vi "Printer Script Trial 1.vi"() -> ()   [LabVIEW 2013]
uses:
  <instrlib>/ZaberTSeries/Public/Utility/Request.ctl
  <instrlib>/ZaberTSeries/ZaberTSeries.lvlib
  <vilib>/MakerHub/LINX/LMH-LINX.lvlib
panel:
  in  "?":T1={"Device Number"=1, "Command"=21, "Data"=-10000, "Response Count"=1} {"Command" items=["Echo"=55, "Home"=1, "Move Absolute"=20, "Move Relative"=21, "Move at Constant Speed"=22, "Renumber"=2, "Restore Settings"=36, "Stop"=23]}
  in  "?":i32=5
  in  "?":T1={"Device Number"=1, "Command"=21, "Data"=-10000, "Response Count"=1} {"Command" items=["Echo"=55, "Home"=1, "Move Absolute"=20, "Move Relative"=21, "Move at Constant Speed"=22, "Renumber"=2, "Restore Settings"=36, "Stop"=23]}
  in  "?":u16
  in  "Select Stage Serial Port \n(COM 10)":refnum<visa-resource-name>
  in  "Select Arduino Serial Port (COM 9)":refnum<visa-resource-name>
  # "Printing Dialogue #1"
  # "Instructions:\n\n1. Select the correct serial ports for the Zaber stage and the Arduino\n\n2. Press the 'Run' arrow at the left of the menu bar. The stage will move forward to accomodate substrate placement. \n\n3. When the substrate has been placed on the stage, click ok in the pop-up dialogue. The stage will then move into place to begin printing. \n\n4. Click OK the 'Begin Printing' pop-up."
  # "Device 1:"
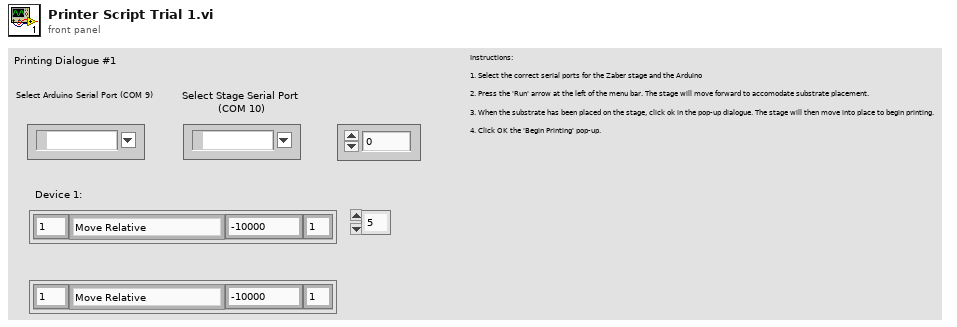
[diagram p1: front panel]
types:
  T1 = typedef "ZaberTSeries.lvlib/Request.ctl" = cluster{"Device Number":u8, "Command":u8, "Data":i32, "Response Count":i32}
  T2 = cluster{"Device Number":u8, "Command":u8, "Data":i32, "Response Count":i32}
  T3 = typedef "LMH-LINX.lvlib/LINX Ref.ctl" = cluster{"Platform":T4, "Interface":T5, "LINX Device Config":T6}
  T4 = typedef "LMH-LINX.lvlib/Platform.ctl" = enum16{"LINX", "myRIO"}
  T5 = typedef "LMH-LINX.lvlib/Interface.ctl" = enum16{"Serial", "TCP"}
  T6 = typedef "LMH-LINX.lvlib/Device.lvlib/LINX Device Config.ctl" = cluster{"Interface":T5, "COM Port":refnum<visa-resource-name>, "TCP Configuration":T7, "Device Family":u8, "Device ID":u8, "Device Name":string, "TCP Ref":refnum<k5>, "Channels":T8}
  T7 = typedef "LMH-LINX.lvlib/Device.lvlib/TCP Config.ctl" = cluster{"IP Address":string, "Port":u16}
  T8 = typedef "LMH-LINX.lvlib/Channels.ctl" = cluster{"DI":u8[], "DO":u8[], "AI":u8[], "AO":u8[], "PWM":u8[], "QE":u8[], "UART":u8[], "I2C 2":u8[], "SPI":u8[], "CAN":u8[], "Servo":u8[], "AI Ref (V)":dbl, "AO Ref (V)":dbl, "AO Resolution (Bits)":u8}
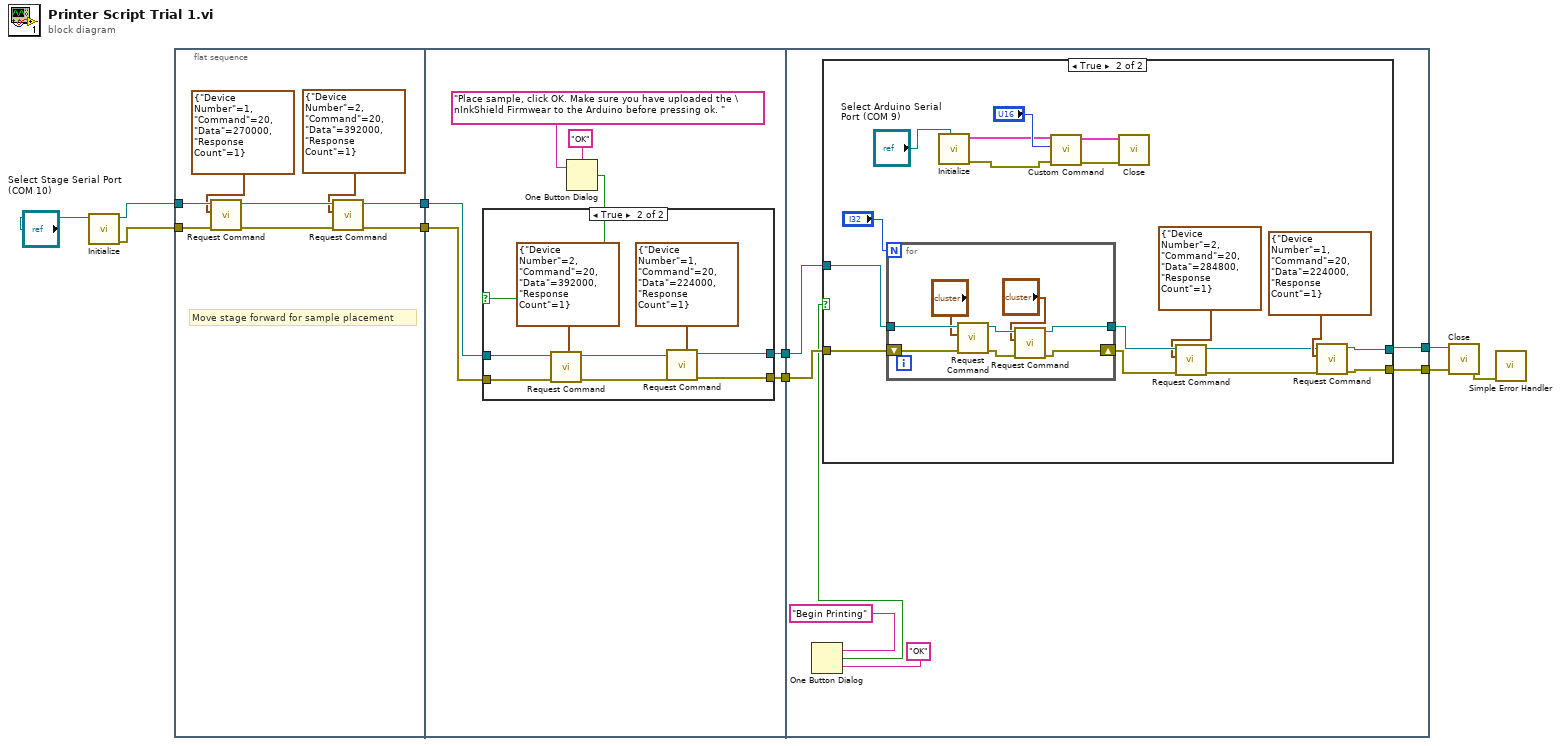
[diagram p0: block diagram]
diagram:
  n1 = call <vilib>:"Initialize.vi"("VISA resource name"="Select Stage Serial Port \n(COM 10)") -> ("error out"=w7:errorcluster, "VISA resource name out"=w8:refnum<visa-resource-name>)  [unwired: 8 in, 1 out]
  n2 = flat-sequence {
    tunnel: w8 -> [w18]
    tunnel: w7 -> [w17]
    tunnel: [w12] -> w6
    tunnel: [w11] -> w5
    tunnel: w6 -> [w22]
    tunnel: w5 -> [w21]
    tunnel: [w20] -> w4
    tunnel: [w19] -> w3
    tunnel: w4 -> [w40]
    tunnel: w3 -> [w39]
    tunnel: [w38] -> w2
    tunnel: [w37] -> w1
    frame #0 {
      # "Move stage forward for sample placement"
      n3 = call <instrlib>:"Request Command.vi"("error in (no error)"=w17, "Request"=T2 {"Device Number"=1, "Command"=20, "Data"=270000, "Response Count"=1}, "VISA resource name"=w18) -> ("error out"=w15:errorcluster, "VISA resource name out"=w16:refnum<visa-resource-name>)  [unwired: 5 in, 2 out]
      n4 = call <instrlib>:"Request Command.vi"("error in (no error)"=w15, "Request"=T2 {"Device Number"=2, "Command"=20, "Data"=392000, "Response Count"=1}, "VISA resource name"=w16) -> ("error out"=w11:errorcluster, "VISA resource name out"=w12:refnum<visa-resource-name>)  [unwired: 5 in, 2 out]
    }
    frame #1 {
      n5 = One Button Dialog(message="Place sample, click OK. Make sure you have uploaded the \nInkShield Firmwear to the Arduino before pressing ok. ", button name ("OK")="OK") -> (true=w23:bool)
      n6 = case shown="True" w23 {
        tunnel: w22 -> [_ w33]
        tunnel: w21 -> [_ w32]
        tunnel: [_ w27] -> w20
        tunnel: [_ w26] -> w19
        frame False {
        }
        frame True {
          n7 = call <instrlib>:"Request Command.vi"("error in (no error)"=w32, "Request"=T2 {"Device Number"=2, "Command"=20, "Data"=392000, "Response Count"=1}, "VISA resource name"=w33) -> ("error out"=w29:errorcluster, "VISA resource name out"=w30:refnum<visa-resource-name>)  [unwired: 5 in, 2 out]
          n8 = call <instrlib>:"Request Command.vi"("error in (no error)"=w29, "Request"=T2 {"Device Number"=1, "Command"=20, "Data"=224000, "Response Count"=1}, "VISA resource name"=w30) -> ("error out"=w26:errorcluster, "VISA resource name out"=w27:refnum<visa-resource-name>)  [unwired: 5 in, 2 out]
        }
      }
    }
    frame #2 {
      n9 = One Button Dialog(message="Begin Printing", button name ("OK")="OK") -> (true=w34:bool)
      n10 = case shown="True" w34 {
        tunnel: [_ w50] -> w38
        tunnel: [_ w49] -> w37
        tunnel: w40 -> [_ w42]
        tunnel: w39 -> [_ w41]
        frame False {
        }
        frame True {
          n11 = for {
            N: "?" -> [_]
            tunnel: w42 -> [w64]
            tunnel: [w59] -> w55
            shift-right: [w61] -> w56
            shift-left: w41 -> [w65]
            n12 = call <instrlib>:"Request Command.vi"("error in (no error)"=w65, "Request"="?", "VISA resource name"=w64) -> ("error out"=w62:errorcluster, "VISA resource name out"=w60:refnum<visa-resource-name>)  [unwired: 5 in, 2 out]
            n13 = call <instrlib>:"Request Command.vi"("error in (no error)"=w62, "Request"="?", "VISA resource name"=w60) -> ("error out"=w61:errorcluster, "VISA resource name out"=w59:refnum<visa-resource-name>)  [unwired: 5 in, 2 out]
          }
          n14 = call <vilib>:"Initialize.vi"("Serial Port"="Select Arduino Serial Port (COM 9)") -> ("Error Out"=w45:errorcluster, "LINX Ref"=w46:T3)  [unwired: 8 in, 1 out]
          n15 = call <vilib>:"Custom Command.vi"("Error In"=w45, "Custom Command Number"="?", "LINX Resource"=w46) -> ("Error Out"=w43:errorcluster, "LINX Resource"=w44:T3)  [unwired: 5 in, 2 out]
          n16 = call <vilib>:"Close.vi"("Error In"=w43, "LINX Resource"=w44) -> ()  [unwired: 8 in, 2 out]
          n17 = call <instrlib>:"Request Command.vi"("error in (no error)"=w56, "Request"=T2 {"Device Number"=2, "Command"=20, "Data"=284800, "Response Count"=1}, "VISA resource name"=w55) -> ("error out"=w51:errorcluster, "VISA resource name out"=w52:refnum<visa-resource-name>)  [unwired: 5 in, 2 out]
          n18 = call <instrlib>:"Request Command.vi"("error in (no error)"=w51, "Request"=T2 {"Device Number"=1, "Command"=20, "Data"=224000, "Response Count"=1}, "VISA resource name"=w52) -> ("error out"=w49:errorcluster, "VISA resource name out"=w50:refnum<visa-resource-name>)  [unwired: 5 in, 2 out]
        }
      }
    }
  }
  n19 = call <vilib>:"Close.vi"("error in (no error)"=w1, "VISA resource name"=w2) -> ("error out"=w9:errorcluster)  [unwired: 8 in, 1 out]
  n20 = call <vilib>:"Simple Error Handler.vi"("error in (no error)"=w9) -> ()  [unwired: 4 in, 5 out]
